vi "dcy05.vi"() -> ()   [LabVIEW 2023]
uses:
  parametertype.ctl
  Public/SECoP-action.ctl
  <vilib>/regexp/Match Regular Expression.xnode
  SECoP.lvlib
panel:
  out "error out":errorcluster
  out "log":string
  in  "DLL path":path=path "D:/shall-repos/shall-labview/64bit"
  in  "stop":bool
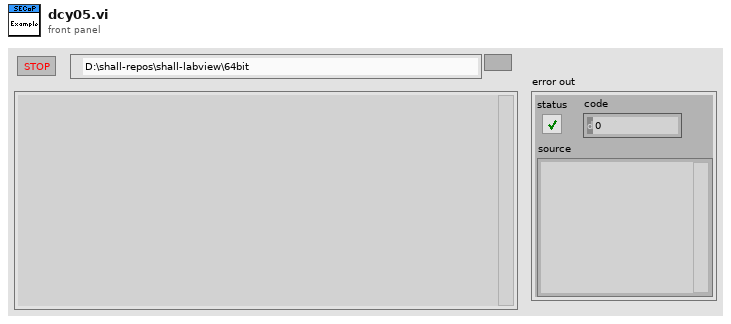
[diagram p1: front panel]
types:
  T1 = typedef "parametertype.ctl" = enum8{"readonly", "readwrite", "command"}
  T2 = cluster{"name":string, "type":T1, "datatype":string, "description":string}[]
  T3 = typedef "SECoP.lvlib/SECoP-libraries.ctl" = cluster{"serverDLL":path, "variantDLL":path, "cleanup_mode":bool, "Context_ID":string}
  T4 = typedef "SECoP.lvlib/SECoP-action.ctl" = enum32{"any action", "read", "change", "do cmd"}
  T5 = cluster{"name":string, "type":T1, "datatype":string, "description":string}
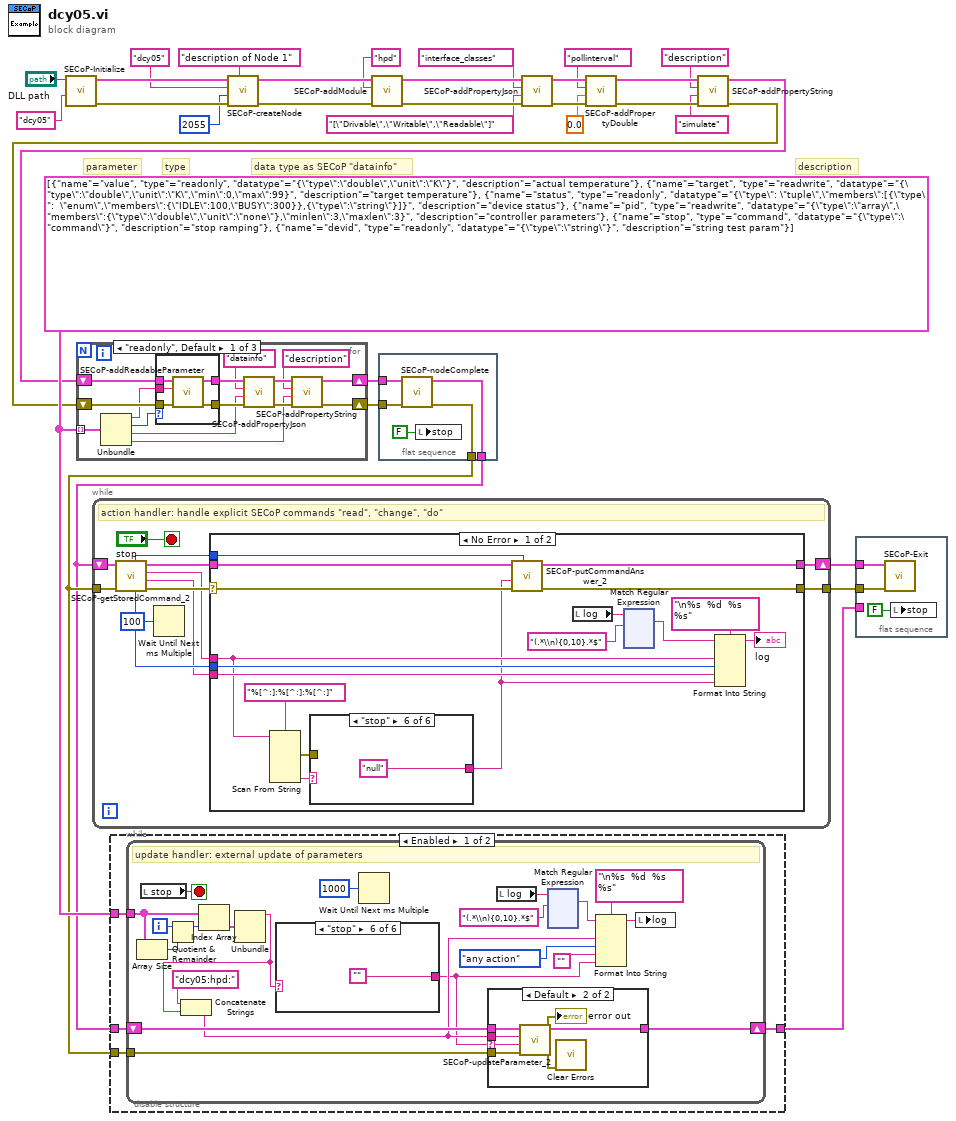
[diagram p0: block diagram]
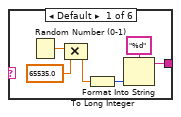
[diagram p3: hidden frame]
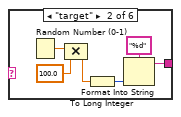
[diagram p4: hidden frame]
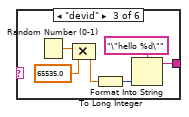
[diagram p5: hidden frame]
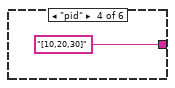
[diagram p6: hidden frame]
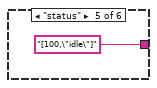
[diagram p7: hidden frame]
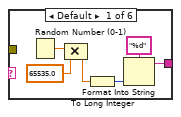
[diagram p9: hidden frame]
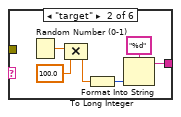
[diagram p10: hidden frame]
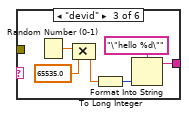
[diagram p11: hidden frame]
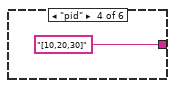
[diagram p12: hidden frame]
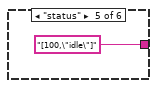
[diagram p13: hidden frame]
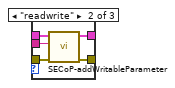
[diagram p15: hidden frame]
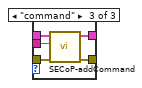
[diagram p16: hidden frame]
diagram:
  w32 = T2 [{"name"="value", "type"=enum."readonly", "datatype"="{\"type\":\"double\",\"unit\":\"K\"}", "description"="actual temperature"}, {"name"="target", "type"=enum."readwrite", "datatype"="{\"type\":\"double\",\"unit\":\"K\",\"min\":0,\"max\":99}", "description"="target temperature"}, {"name"="status", "type"=enum."readonly", "datatype"="{\"type\": \"tuple\",\"members\":[{\"type\":  \"enum\",\"members\":{\"IDLE\":100,\"BUSY\":300}},{\"type\":\"string\"}]}", "description"="device status"}, {"name"="pid", "type"=enum."readwrite", "datatype"="{\"type\":\"array\",\"members\":{\"type\":\"double\",\"unit\":\"none\"},\"minlen\":3,\"maxlen\":3}", "description"="controller parameters"}, {"name"="stop", "type"=enum."command", "datatype"="{\"type\":\"command\"}", "description"="stop ramping"}, {"name"="devid", "type"=enum."readonly", "datatype"="{\"type\":\"string\"}", "description"="string test param"}]
  # "description"
  # "data type as SECoP \"datainfo\""
  # "type"
  # "parameter"
  n1 = call "SECoP-Initialize.vi"("Context ID (in)"="dcy05", "DLL path (in)"="DLL path") -> ("error out"=w26:errorcluster, "DLL path (out)"=w27:T3)  [unwired: 8 in]
  n2 = while {
    shift-right: [w44] -> w15
    shift-left: w5 -> [w42]
    tunnel: w31 -> [w41]
    tunnel: [w34] -> w14
    stop <- "stop" stop-if-true
    # "action handler: handle explicit SECoP commands \"read\", \"change\", \"do\""
    n3 = call "SECoP-getStoredCommand_2.vi"("error in (no error)"=w41, "DLL path (in)"=w42) -> ("error out"=w39:errorcluster, "arguments/setvalue"=w35:string, "command/parameter path"=w36:string, "DLL path (out)"=w40:T3, "action"=w37:T4, "command id"=w38:u64)  [unwired: 4 in]
    n4 = Wait Until Next ms Multiple(millisecond multiple=u32 100) -> ()  [unwired: 1 out]
    n5 = case shown="No Error" w39 {
      selector: w39 -> [w61 w200]
      tunnel: w40 -> [w60 w201]
      tunnel: [w59 w201] -> w44
      tunnel: w38 -> [w58 _]
      tunnel: w36 -> [w49 _]
      tunnel: w35 -> [w55 _]
      tunnel: w37 -> [w56 _]
      tunnel: [w57 w200] -> w34
      frame No Error {
        n6 = Scan From String(format string="%[^:]:%[^:]:%[^:]", input string=w49) -> (error out=w46:errorcluster, output 3=w48:string)  [unwired: 7 in, 2 out]
        n7 = case shown="\"stop\"" w48 {
          tunnel: [w62 w68 w74 "[10,20,30]" "[100,\"idle\"]" "null"] -> w47
          tunnel: w46 -> [_ _ _ _ _ _]
          frame Default {
            n8 = Random Number (0-1)() -> (number: 0 to 1=w64:dbl)
            n9 = Compound Arithmetic op=MULTIPLY(w64, 65535.0 ("value")) -> (w66:dbl)
            n10 = To Long Integer(number=w66) -> (32bit integer=w67:i32)
            n11 = Format Into String(format string="%d", w67) -> (resulting string=w62:string)  [unwired: 2 in, 1 out]
          }
          frame "target" {
            n12 = Random Number (0-1)() -> (number: 0 to 1=w70:dbl)
            n13 = Compound Arithmetic op=MULTIPLY(w70, 100.0 ("value")) -> (w72:dbl)
            n14 = To Long Integer(number=w72) -> (32bit integer=w73:i32)
            n15 = Format Into String(format string="%d", w73) -> (resulting string=w68:string)  [unwired: 2 in, 1 out]
          }
          frame "devid" {
            n16 = Random Number (0-1)() -> (number: 0 to 1=w76:dbl)
            n17 = Compound Arithmetic op=MULTIPLY(w76, 65535.0 ("value")) -> (w78:dbl)
            n18 = To Long Integer(number=w78) -> (32bit integer=w79:i32)
            n19 = Format Into String(format string="\"hello %d\"", w79) -> (resulting string=w74:string)  [unwired: 2 in, 1 out]
          }
          frame "pid" {
          }
          frame "status" {
          }
          frame "stop" {
          }
        }
        n20 = call "SECoP-putCommandAnswer_2.vi"("command id"=w58, "error in (no error)"=w61, "value"=w47, "DLL path (in)"=w60) -> ("error out"=w57:errorcluster, "DLL path (out)"=w59:T3)  [unwired: 6 in]
        n21 = local read "log"() -> (w52:string)
        n22 = xnode "Match Regular Expression"("input string"=w52, "regular expression"="(.*\\n){0,10}.*$") -> ("whole match"=w53:string)  [unwired: 4 in, 4 out]
        n23 = Format Into String(format string="\n%s  %d  %s  %s", initial string=w53, w49, w56, w55, w47) -> (resulting string=→"log":string)  [unwired: 1 in, 1 out]
      }
      frame Error {
      }
    }
  }
  n24 = disable-structure shown="Enabled" {
    disable-tunnel: w31 -> [w205 _]
    disable-tunnel: w32 -> [w204 _]
    disable-tunnel: w5 -> [w203 w372]
    disable-tunnel: [w202 w372] -> w4
    frame Enabled {
      n25 = while {
        tunnel: w205 -> [w207]
        shift-right: [w224] -> w202
        shift-left: w203 -> [w225]
        tunnel: w204 -> [w217]
        i -> [w219]
        stop <- w226 stop-if-true
        # "update handler: external update of parameters"
        n26 = Array Size(array=w217) -> (size(s)=w220:i32)
        n27 = local read "stop"() -> (w226:bool)
        n28 = Quotient & Remainder(x=w219, y=w220) -> (x-y*floor(x/y)=w221:i32)  [unwired: 1 out]
        n29 = Index Array(array=w217, index=w221) -> (element=w218:T5)
        n30 = Unbundle(w218) -> ("name"=w208:string)  [unwired: 3 out]
        n31 = Concatenate Strings("dcy05:hpd:" ("string"), w208) -> (w212:string)
        n32 = case shown="\"stop\"" w208 {
          tunnel: [w234 w240 w246 "[10,20,30]" "[100,\"idle\"]" ""] -> w206
          frame Default {
            n33 = Random Number (0-1)() -> (number: 0 to 1=w236:dbl)
            n34 = Compound Arithmetic op=MULTIPLY(w236, 65535.0 ("value")) -> (w238:dbl)
            n35 = To Long Integer(number=w238) -> (32bit integer=w239:i32)
            n36 = Format Into String(format string="%d", w239) -> (resulting string=w234:string)  [unwired: 2 in, 1 out]
          }
          frame "target" {
            n37 = Random Number (0-1)() -> (number: 0 to 1=w242:dbl)
            n38 = Compound Arithmetic op=MULTIPLY(w242, 100.0 ("value")) -> (w244:dbl)
            n39 = To Long Integer(number=w244) -> (32bit integer=w245:i32)
            n40 = Format Into String(format string="%d", w245) -> (resulting string=w240:string)  [unwired: 2 in, 1 out]
          }
          frame "devid" {
            n41 = Random Number (0-1)() -> (number: 0 to 1=w248:dbl)
            n42 = Compound Arithmetic op=MULTIPLY(w248, 65535.0 ("value")) -> (w250:dbl)
            n43 = To Long Integer(number=w250) -> (32bit integer=w251:i32)
            n44 = Format Into String(format string="\"hello %d\"", w251) -> (resulting string=w246:string)  [unwired: 2 in, 1 out]
          }
          frame "pid" {
          }
          frame "status" {
          }
          frame "stop" {
          }
        }
        n45 = Wait Until Next ms Multiple(millisecond multiple=u32 1000) -> ()  [unwired: 1 out]
        n46 = case shown="Default" w206 {
          selector: w206 -> [_ w228]
          tunnel: w225 -> [w227 w233]
          tunnel: [w227 w232] -> w224
          tunnel: w212 -> [_ w231]
          tunnel: w207 -> [_ w230]
          frame "" {
          }
          frame Default {
            n47 = call "SECoP-updateParameter_2.vi"("error in (no error)"=w230, "value"=w228, "parameter name"=w231, "DLL path (in)"=w233) -> ("error out"=w229:errorcluster, "DLL path (out)"=w232:T3)  [unwired: 6 in]
            "error out" <- w229
            n48 = call <vilib>:"Clear Errors.vi"("error in (no error)"=w229) -> ()  [unwired: 5 in, 2 out]
          }
        }
        n49 = local read "log"() -> (w216:string)
        n50 = xnode "Match Regular Expression"("input string"=w216, "regular expression"="(.*\\n){0,10}.*$") -> ("whole match"=w215:string)  [unwired: 4 in, 4 out]
        n51 = Format Into String(format string="\n%s  %d  %s  %s", initial string=w215, w212, SECoP-action."any action" ("input 2"), "", w206) -> (resulting string=w209:string)  [unwired: 1 in, 1 out]
        n52 = local write "log"(w209) -> ()
      }
    }
    frame Disabled {
    }
  }
  n53 = call "SECoP-createNode.vi"("description"="description of Node 1", "error in (no error)"=w26, "TCP port"=u16 2055, "node id"="dcy05" ("id"), "DLL path (in)"=w27) -> ("error out"=w21:errorcluster, "DLL path (out)"=w25:T3)  [unwired: 5 in]
  n54 = call "SECoP-addModule.vi"("error in (no error)"=w21, "module name"="hpd" ("name"), "DLL path (in)"=w25) -> ("error out"=w18:errorcluster, "DLL path (out)"=w19:T3)  [unwired: 7 in]
  n55 = flat-sequence {
    tunnel: w7 -> [w376]
    tunnel: w6 -> [w375]
    tunnel: [w373] -> w5
    tunnel: [w374] -> w31
    frame #0 {
      n56 = call "SECoP-nodeComplete.vi"("error in (no error)"=w375, "DLL path (in)"=w376) -> ("error out"=w374:errorcluster, "DLL path (out)"=w373:T3)  [unwired: 8 in]
      n57 = local write "stop"(FALSE) -> ()
    }
  }
  n58 = call "SECoP-addPropertyJson.vi"("error in (no error)"=w18, "property value"="[\"Drivable\",\"Writable\",\"Readable\"]" ("name"), "property name"="interface_classes" ("name"), "DLL path (in)"=w19) -> ("error out"=w10:errorcluster, "DLL path (out)"=w11:T3)  [unwired: 6 in]
  n59 = call "SECoP-addPropertyDouble.vi"("error in (no error)"=w10, "property value"=0.0, "property name"="pollinterval", "DLL path (in)"=w11) -> ("error out"=w30:errorcluster, "DLL path (out)"=w29:T3)  [unwired: 6 in]
  n60 = call "SECoP-addPropertyString.vi"("error in (no error)"=w30, "property value"="simulate" ("name"), "property name"="description" ("name"), "DLL path (in)"=w29) -> ("error out"=w2:errorcluster, "DLL path (out)"=w3:T3)  [unwired: 6 in]
  n61 = for {
    tunnel: w32 -> [w380] mode=indexing
    shift-right: [w379] -> w7
    shift-left: w3 -> [w389]
    shift-right: [w378] -> w6
    shift-left: w2 -> [w388]
    n62 = Unbundle(w380) -> ("name"=w381:string, "type"=w390:T1, "datatype"=w382:string, "description"=w383:string)
    n63 = case shown="\"readonly\", Default" w390 {
      tunnel: w381 -> [w395 w402 w407]
      tunnel: w389 -> [w397 w401 w406]
      tunnel: [w396 w400 w405] -> w387
      tunnel: [w393 w398 w403] -> w386
      tunnel: w388 -> [w394 w399 w404]
      frame "readonly", Default {
        n64 = call "SECoP-addReadableParameter.vi"("error in (no error)"=w394, "parameter name"=w395, "DLL path (in)"=w397) -> ("error out"=w393:errorcluster, "DLL path (out)"=w396:T3)  [unwired: 7 in]
      }
      frame "readwrite" {
        n65 = call "SECoP-addWritableParameter.vi"("error in (no error)"=w399, "parameter name"=w402, "DLL path (in)"=w401) -> ("error out"=w398:errorcluster, "DLL path (out)"=w400:T3)  [unwired: 7 in]
      }
      frame "command" {
        n66 = call "SECoP-addCommand.vi"("error in (no error)"=w404, "command name"=w407, "DLL path (in)"=w406) -> ("error out"=w403:errorcluster, "DLL path (out)"=w405:T3)  [unwired: 7 in]
      }
    }
    n67 = call "SECoP-addPropertyJson.vi"("error in (no error)"=w386, "property value"=w382, "property name"="datainfo" ("name"), "DLL path (in)"=w387) -> ("error out"=w391:errorcluster, "DLL path (out)"=w392:T3)  [unwired: 6 in]
    n68 = call "SECoP-addPropertyString.vi"("error in (no error)"=w391, "property value"=w383, "property name"="description" ("name"), "DLL path (in)"=w392) -> ("error out"=w378:errorcluster, "DLL path (out)"=w379:T3)  [unwired: 6 in]
  }
  n69 = flat-sequence {
    tunnel: w15 -> [w409]
    tunnel: w14 -> [w408]
    tunnel: w4 -> [_]
    frame #0 {
      n70 = call "SECoP-Exit.vi"("error in (no error)"=w408, "DLL path (in)"=w409) -> ()  [unwired: 9 in, 1 out]
      n71 = local write "stop"(FALSE) -> ()
    }
  }
